vi "USB2XXX_LINEX_MasterSimpleWriteReadTest.vi"() -> ()   [LabVIEW 2010]
panel:
  in  "CeckType":u8(ring) items=["标准校验", "增强校验"]
  in  "pData Wite":u8[](array[numeric])=[0, 0, 0, 0, 0, 0, 0, 0] format="%x"
  in  "stop":bool
  out "pData Read":u8[](array[numeric]) format="%x"
  out "Readed Data Num":i32
  out "Read Data(Hex)":string
  in  "Read Data ID":u8=61 format="%x"
  in  "Write Data ID":u8=60 format="%x"
  in  "BaudRate":u32=19200
  in  "Channel Index":u8(ring) items=["LIN1", "LIN2"]
  in  "Device Index":i32(ring) items=["0", "1", "2", "3", "4", "5"]
  # "波特率一定要设置，否则程序可能出错"
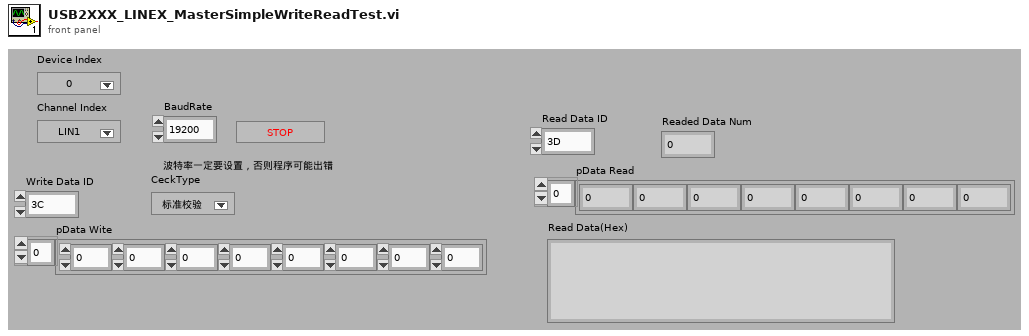
[diagram p1: front panel]
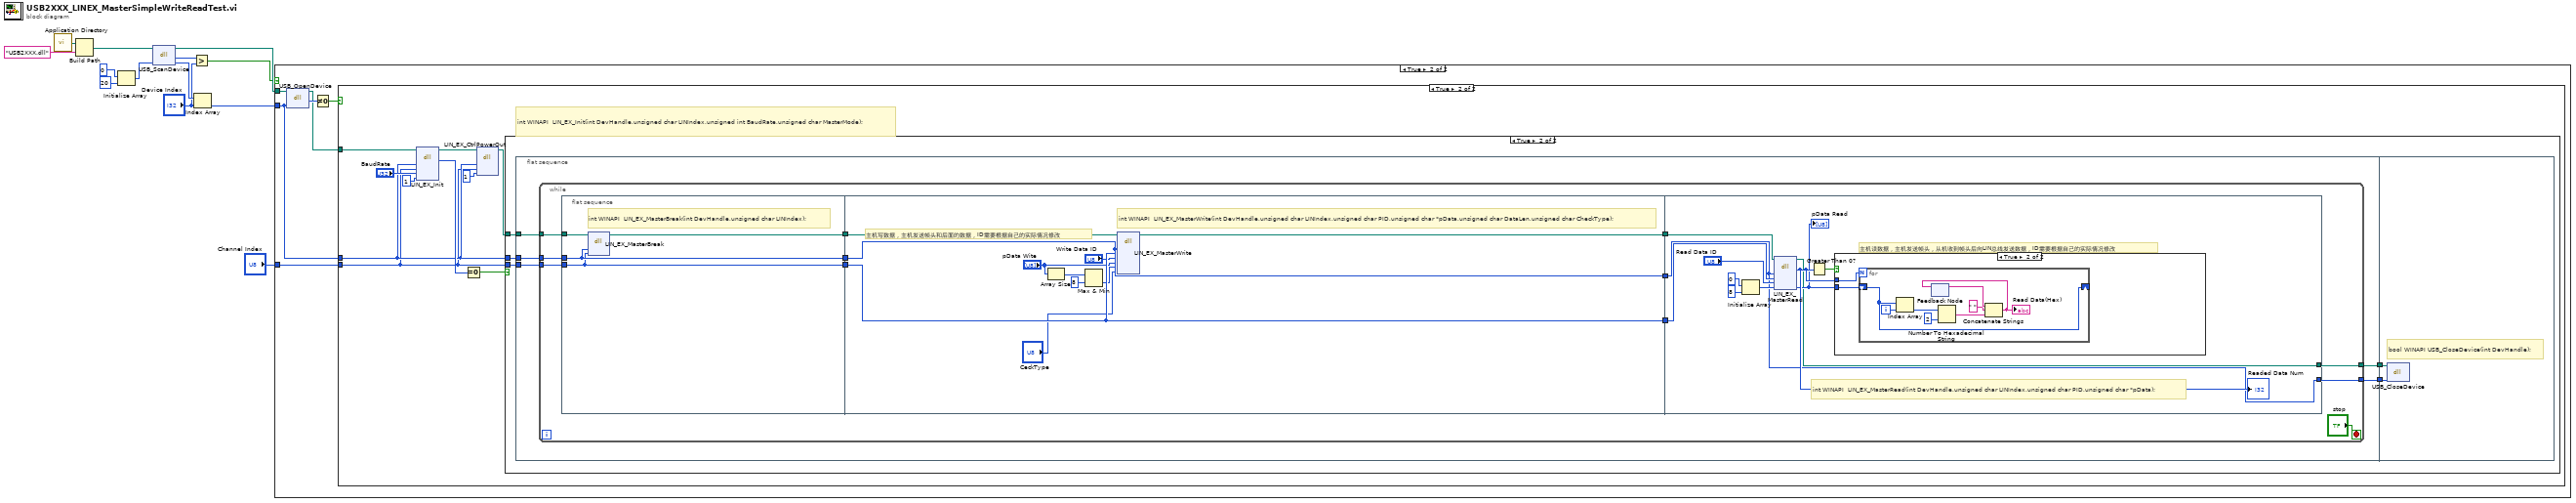
[diagram p0: block diagram]
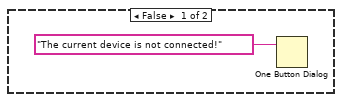
[diagram p2: hidden frame]
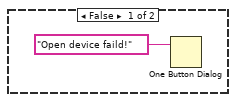
[diagram p3: hidden frame]
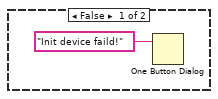
[diagram p4: hidden frame]
diagram:
  n1 = call <vilib>:"Application Directory.vi"() -> ("Application Directory"=w5:path)
  n2 = Build Path(base path=w5, name or relative path="USB2XXX.dll") -> (appended path=w4:path)
  n3 = Initialize Array(0, 20 ("dimension size")) -> (w11:i32[])
  n4 = dll-call lib="E:/OtherWork/STM32/USB2XXX_Example/examples/Labview/PublicFiles/USB2XXX.dll" fn="USB_ScanDevice"(path in=w4, "pDevNum"=w11) -> (path out=w9:path, "return type"=w3:i32, "pDevNum"=w10:i32[])  [unwired: 2 in, 1 out]
  n5 = Greater?(x=w3, y="Device Index") -> (0:w1:bool)
  n6 = Index Array(array=w10, index="Device Index") -> (element=w8:i32)
  n7 = case shown="True" w1 {
    tunnel: w9 -> [_ w20]
    tunnel: w8 -> [_ w16]
    tunnel: "Channel Index" -> [_ w15]
    frame False {
      n8 = One Button Dialog(message="The current device is not connected!") -> ()  [unwired: 1 in, 1 out]
    }
    frame True {
      n9 = dll-call lib="E:/OtherWork/STM32/USB2XXX_Example/examples/Labview/PublicFiles/USB2XXX.dll" fn="USB_OpenDevice"(path in=w20, "DevIndex"=w16) -> (path out=w17:path, "return type"=w19:u8)  [unwired: 3 in, 1 out]
      n10 = Not Equal To 0?(x=w19) -> (x != 0?=w18:bool)
      n11 = case shown="True" w18 {
        tunnel: w17 -> [_ w29]
        tunnel: w16 -> [_ w24]
        tunnel: w15 -> [_ w23]
        frame False {
          n12 = One Button Dialog(message="Open device faild!") -> ()  [unwired: 1 in, 1 out]
        }
        frame True {
          # "int WINAPI  LIN_EX_Init(int DevHandle,unsigned char LINIndex,unsigned int BaudRate,unsigned char MasterMode);"
          n13 = dll-call lib="E:/OtherWork/STM32/USB2XXX_Example/examples/Labview/PublicFiles/USB2XXX.dll" fn="LIN_EX_Init"(path in=w29, "DevHandle"=w24, "LINIndex"=w23, "BaudRate"="BaudRate", "MasterMode"=u8 1) -> (path out=w25:path, "return type"=w28:i32)  [unwired: 6 in, 1 out]
          n14 = Equal To 0?(x=w28) -> (x = 0?=w27:bool)
          n15 = dll-call lib="E:/Projects/USB2XXX/trunk/USB2XXX/USB2XXX/vs2010/Release/USB2XXX.*" fn="LIN_EX_CtrlPowerOut"(path in=w25, "DevHandle"=w24, "LINIndex"=w23, "VbatValue"=u8 1 ("State")) -> (path out=w26:path)  [unwired: 6 in, 1 out]
          n16 = case shown="True" w27 {
            tunnel: w26 -> [_ w37]
            tunnel: w24 -> [_ w36]
            tunnel: w23 -> [_ w35]
            frame False {
              n17 = One Button Dialog(message="Init device faild!") -> ()  [unwired: 1 in, 1 out]
            }
            frame True {
              n18 = flat-sequence {
                tunnel: w37 -> [w42]
                tunnel: w36 -> [w41]
                tunnel: w35 -> [w40]
                tunnel: [w39] -> w34
                tunnel: [w38] -> w33
                tunnel: w34 -> [w91]
                tunnel: w33 -> [w90]
                frame #0 {
                  n19 = while {
                    tunnel: w42 -> [w51]
                    tunnel: w41 -> [w50]
                    tunnel: w40 -> [w49]
                    tunnel: [w44] -> w39
                    tunnel: [w43] -> w38
                    stop <- "stop" stop-if-true
                    n20 = flat-sequence {
                      tunnel: w51 -> [w58]
                      tunnel: w50 -> [w56]
                      tunnel: w49 -> [w55]
                      tunnel: [w55] -> w47
                      tunnel: [w56] -> w46
                      tunnel: [w57] -> w45
                      tunnel: [w68] -> w54
                      tunnel: [w67] -> w53
                      tunnel: [w66] -> w52
                      tunnel: w47 -> [w66]
                      tunnel: w46 -> [w67]
                      tunnel: w45 -> [w64]
                      tunnel: w54 -> [w79]
                      tunnel: w53 -> [w70]
                      tunnel: w52 -> [w78]
                      tunnel: [w70] -> w44
                      tunnel: [w69] -> w43
                      frame #0 {
                        # "int WINAPI  LIN_EX_MasterBreak(int DevHandle,unsigned char LINIndex);"
                        n21 = dll-call lib="E:/Projects/USB2XXX/trunk/USB2XXX/USB2XXX/vs2010/Release/USB2XXX.*" fn="LIN_EX_MasterBreak"(path in=w58, "DevHandle"=w56, "LINIndex"=w55) -> (path out=w57:path)  [unwired: 5 in, 1 out]
                      }
                      frame #1 {
                        # "主机写数据，主机发送帧头和后面的数据，ID需要根据自己的实际情况修改"
                        # "int WINAPI  LIN_EX_MasterWrite(int DevHandle,unsigned char LINIndex,unsigned char PID,unsigned char *pData,unsigned char DataLen,unsigned char CheckType);"
                        n22 = Array Size(array="pData Wite") -> (size(s)=w63:i32)
                        n23 = Max & Min(x=w63, y=8) -> (min(x,y)=w61:i32)  [unwired: 1 out]
                        n24 = dll-call lib="E:/OtherWork/STM32/USB2XXX_Example/sdk/api/Labview/USB2XXX.*" fn="LIN_EX_MasterWrite"(path in=w64, "DevHandle"=w67, "LINIndex"=w66, "PID"="Write Data ID", "pData"="pData Wite", "DataLen"=w61, "CheckType"="CeckType") -> (path out=w68:path)  [unwired: 9 in, 1 out]
                      }
                      frame #2 {
                        # "主机读数据，主机发送帧头，从机收到帧头后向LIN总线发送数据，ID需要根据自己的实际情况修改"
                        # "int WINAPI  LIN_EX_MasterRead(int DevHandle,unsigned char LINIndex,unsigned char PID,unsigned char *pData);"
                        n25 = Initialize Array(u8 0 ("element"), 8 ("dimension size")) -> (w74:u8[])
                        n26 = dll-call lib="E:/OtherWork/STM32/USB2XXX_Example/sdk/api/Labview/USB2XXX.*" fn="LIN_EX_MasterRead"(path in=w79, "DevHandle"=w70, "LINIndex"=w78, "PID"="Read Data ID", "pData"=w74) -> (path out=w69:path, "return type"=w72:i32, "pData"=w71:u8[])  [unwired: 5 in, 1 out]
                        "Readed Data Num" <- w72
                        "pData Read" <- w71
                        n27 = Greater Than 0?(x=w72) -> (x > 0?=w76:bool)
                        n28 = case shown="True" w76 {
                          tunnel: w72 -> [_ w81]
                          tunnel: w71 -> [_ w80]
                          frame False {
                          }
                          frame True {
                            n29 = for {
                              N: w81 -> [_]
                              shift-right: [w82] -> _
                              shift-left: w80 -> [w82]
                              i -> [w89]
                              n30 = Index Array(array=w82, index=w89) -> (element=w88:u8)
                              n31 = feedback #1() -> (w86:string)  [unwired: 1 in]
                              n32 = Number To Hexadecimal String(1:i16 2 ("width (-)"), 2:w88) -> (0:w84:string)
                              n33 = Concatenate Strings(w86, " " ("string"), w84) -> (w83:string)
                              "Read Data(Hex)" <- w83
                              n34 = feedback-in #1(w83) -> ()
                            }
                          }
                        }
                      }
                    }
                  }
                }
                frame #1 {
                  # "bool WINAPI USB_CloseDevice(int DevHandle);"
                  n35 = dll-call lib="E:/Projects/USB2XXX/trunk/USB2XXX/USB2XXX/vs2010/Release/USB2XXX.*" fn="USB_CloseDevice"(path in=w90, "DevHandle"=w91) -> ()  [unwired: 4 in, 2 out]
                }
              }
            }
          }
        }
      }
    }
  }
